vi "TTA_MATLAB_Tile_RFPAL_Load_Cal_Freq.vi"(0 "Channels":string[](array[combo]), 1 "Frequency3":dbl, 2 "Frequency4":dbl, 5 "Frequency ID":i32, 7 "Frequency1":dbl, 9 "Frequency2":dbl, 11 "error in":errorcluster) -> (4 "Success":bool, 6 "TileSuccessComm":bool[](array[boolean]), 15 "error out":errorcluster)   [LabVIEW 2016]
panel:
  out "TileSuccessOp":bool[](array[boolean])
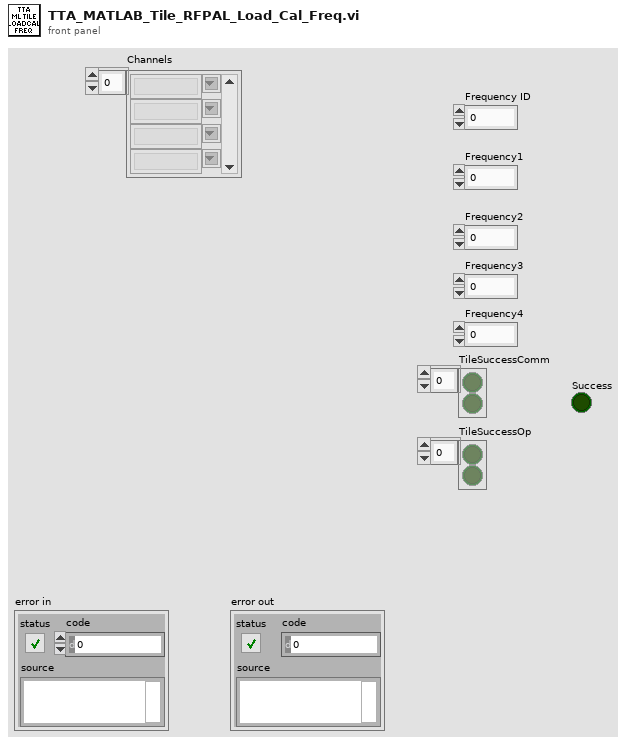
[diagram p1: front panel]
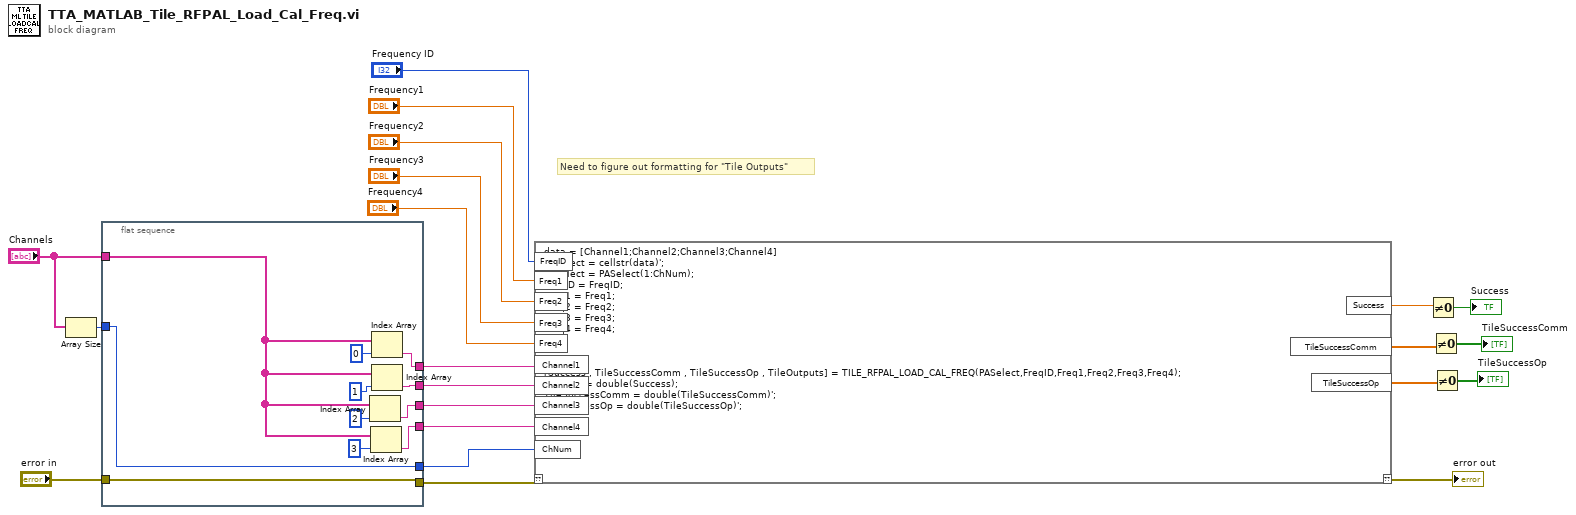
[diagram p0: block diagram]
diagram:
  # "Need to figure out formatting for \"Tile Outputs\""
  n1 = Array Size(array="Channels") -> (size(s)=w19:i32)
  n2 = flat-sequence {
    tunnel: "error in" -> [w32]
    tunnel: [w31] -> w18
    tunnel: w19 -> [w25]
    tunnel: [w32] -> w17
    tunnel: "Channels" -> [w24]
    tunnel: [w28] -> w5
    tunnel: [w26] -> w4
    tunnel: [w25] -> w3
    tunnel: [w22] -> w2
    frame #0 {
      n3 = Index Array(array=w24, index=2) -> (element=w26:string)
      n4 = Index Array(array=w24, index=3) -> (element=w22:string)
      n5 = Index Array(array=w24, index=0) -> (element=w31:string)
      n6 = Index Array(array=w24, index=1) -> (element=w28:string)
    }
  }
  n7 = script code="data = [Channel1;Channel2;Channel3;Channel4]\nPASelect = cellstr(data)';\nPASelect = PASelect(1:ChNum);\nFreqID = FreqID;\nFreq1 = Freq1;\nFreq2 = Freq2;\nFreq3 = Freq3;\nFreq4 = Freq4;\n\n\n\n[Success , TileSuccessComm , TileSuccessOp , TileOutputs] = TILE_RFPAL_LOAD_CAL_FREQ(PASelect,FreqID,Freq1,Freq2,Freq3,Freq4);\nSuccess = double(Success);\nTileSuccessComm = double(TileSuccessComm)';\nTileSuccessOp = double(TileSuccessOp)';"("??"=w17, "Channel1"=w18, "FreqID"="Frequency ID", "Freq1"="Frequency1", "Freq2"="Frequency2", "Freq3"="Frequency3", "Freq4"="Frequency4", "Channel2"=w5, "Channel3"=w4, "Channel4"=w2, "ChNum"=w3) -> ("??"=→"error out":errorcluster, "Success"=w10:dbl, "TileSuccessComm"=w9:dbl[], "TileSuccessOp"=w8:dbl[])
  n8 = Not Equal To 0?(x=w10) -> (x != 0?=→"Success":bool)
  n9 = Not Equal To 0?(x=w9) -> (x != 0?=→"TileSuccessComm":bool[])
  n10 = Not Equal To 0?(x=w8) -> (x != 0?=→"TileSuccessOp":bool[])
